vi "New Sequence Execution.vi"(8 "error in (no error)":errorcluster, 11 "teststand-api in":refnum<class "teststand-api.lvclass">) -> (0 "error out":errorcluster, 3 "teststand-api out":refnum<class "teststand-api.lvclass">)   [LabVIEW 2014, in "teststand-api.lvlib" / "teststand-api.lvclass"]
uses:
  teststand-api.lvclass
  teststand-api.lvclass/teststand-api.ctl
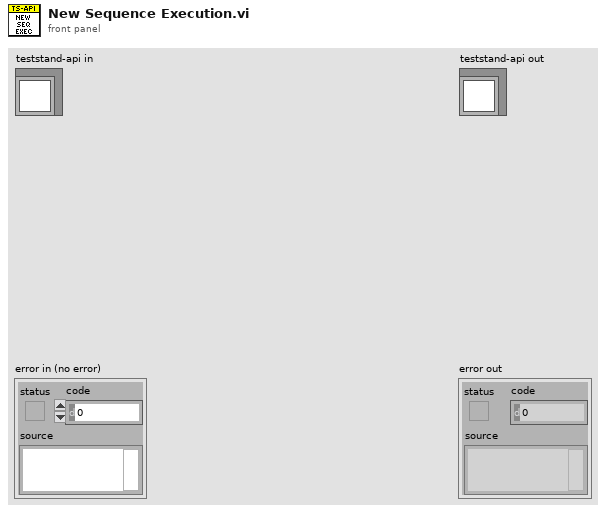
[diagram p1: front panel]
types:
  T1 = typedef "teststand-api.lvlib/teststand-api.lvclass/Model Run Mode--enum.ctl" = enum16{"Test UUTs", "Single Pass"}
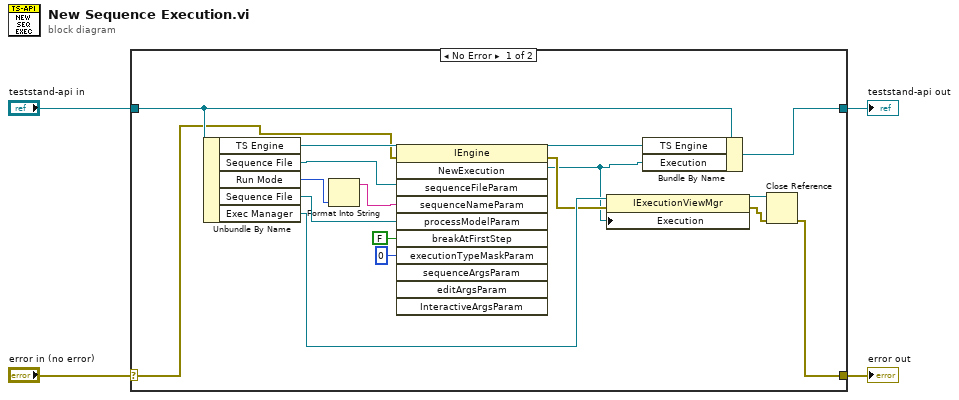
[diagram p0: block diagram]
diagram:
  n1 = case shown="No Error" "error in (no error)" {
    selector: "error in (no error)" -> [w9 w23]
    tunnel: [w5 w23] -> w3
    tunnel: [w19 w22] -> w1
    tunnel: "teststand-api in" -> [w20 w22]
    frame No Error {
      n2 = Unbundle By Name(w20) -> ("TS Engine"=w21:refnum<k7>, "Sequence File"=w18:refnum<k7>, "Run Mode"=w17:T1, "Sequence File"=w15:refnum<k7>, "Exec Manager"=w11:refnum<k7>)
      n3 = Format Into String(w17) -> (resulting string=w16:string)  [unwired: 3 in, 1 out]
      n4 = invoke class="IEngine" method="NewExecution"(reference=w21, error in=w9, "sequenceFileParam"=w18, "sequenceNameParam"=w16, "processModelParam"=w15, "breakAtFirstStep"=FALSE, "executionTypeMaskParam"=0) -> (reference out=w12:refnum<k7>, error out=w10:errorcluster, "NewExecution"=w8:refnum<k7>)  [unwired: 4 in, 8 out]
      n5 = property class="IExecutionViewMgr"(reference=w11, error in=w10, "Execution"=w8) -> (reference out=w7:refnum<k7>, error out=w6:errorcluster)
      n6 = Bundle By Name(cluster=w20, "TS Engine"=w12, "Execution"=w8) -> (w19:refnum<class "teststand-api.lvclass">)
      n7 = Close Reference(reference=w7, error in (no error)=w6) -> (error out=w5:errorcluster)
    }
    frame Error {
    }
  }
  "error out" <- w3
  "teststand-api out" <- w1
